vi "G4SubTemplate_Singleton_4x4x4_Init.vi"(8 "Error In":errorcluster, 11 "reference in":refnum<class "G4SubTemplate_Singleton_4x4x4.lvclass"> caption="This control should only be used when\na sub class is inheriting this class") -> (0 "Error Out":errorcluster, 3 "reference out":refnum<class "G4SubTemplate_Singleton_4x4x4.lvclass"> caption="This indicator should only be used when\na sub class is inheriting this class")   [LabVIEW 2020, in "G4SubTemplate_Singleton_4x4x4.lvclass"]
uses:
  <resource>/Framework/Providers/Open_GDS/ClassProviders/Provider_EndevoGOOP400/Templates/G4SubTemplate_Singleton_4x4x4/G4SubTemplate_Singleton_4x4x4.lvclass
  C:/Program Files (x86)/National Instruments/LabVIEW 2020/resource/Framework/Providers/Open_GDS/ClassProviders/Provider_EndevoGOOP400/Templates/G4BaseTemplate_Singleton_4x4x4/G4BaseTemplate_Singleton_4x4x4.lvclass
  <resource>/Framework/Providers/Open_GDS/ClassProviders/Provider_EndevoGOOP400/Templates/G4BaseTemplate_Singleton_4x4x4/G4BaseTemplate_Singleton_4x4x4.lvclass
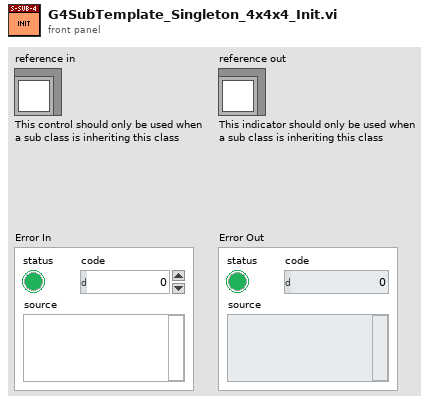
[diagram p1: front panel]
types:
  T1 = typedef "G4SubTemplate_Singleton_4x4x4.lvclass/ObjectAttributes.ctl" = cluster{"Attribute1":dbl}
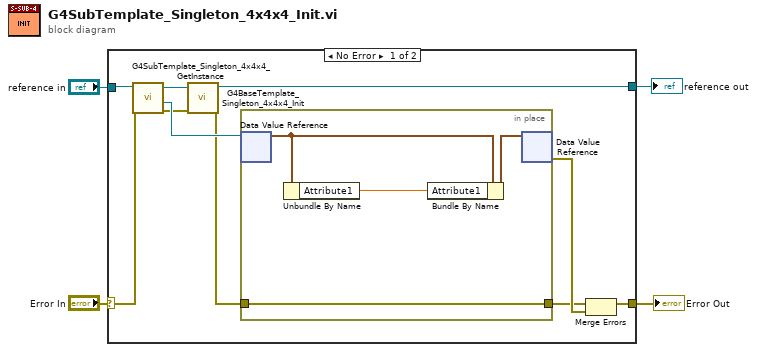
[diagram p0: block diagram]
diagram:
  n1 = case shown="No Error" "Error In" {
    selector: "Error In" -> [w11 w20]
    tunnel: [w12 w20] -> w3
    tunnel: "reference in" -> [w8 w19]
    tunnel: [w7 w19] -> w1
    frame No Error {
      n2 = call <resource>:"G4SubTemplate_Singleton_4x4x4_GetInstance.vi"("error in"=w11, "reference in"=w8) -> ("error out"=w10:errorcluster, "DVRRefOut"=w14:refnum<data-value>, "reference out"=w9:refnum<class "G4SubTemplate_Singleton_4x4x4.lvclass">)  [unwired: 5 in, 2 out]
      n3 = call <resource>:"G4BaseTemplate_Singleton_4x4x4_Init.vi"("Error In"=w10, "reference in"=w9) -> ("Error Out"=w6:errorcluster, "reference out"=w7:refnum<class "G4SubTemplate_Singleton_4x4x4.lvclass">)  [unwired: 8 in]
      n4 = in-place {
        in-place-border: w6 -> [w15]
        in-place-border: [w15] -> w5
        n5 = in-place-dvr #1(w14) -> (w17:T1)  [unwired: 1 out]
        n6 = Unbundle By Name(w17) -> ("Attribute1"=w16:dbl)
        n7 = Bundle By Name(cluster=w17, "Attribute1"=w16) -> (w18:T1)
        n8 = in-place-dvr #1(w18) -> (w13:errorcluster)  [unwired: 1 out]
      }
      n9 = Merge Errors(w5, w13) -> (w12:errorcluster)
    }
    frame Error {
    }
  }
  "Error Out" <- w3
  "reference out" <- w1
